vi "Frameremap.vi"(8 "FH":dbl, 9 "FW":dbl, 10 "FO Z":dbl, 11 "FO X":dbl) -> (0 "FH":dbl, 1 "FW":dbl, 2 "Z Origin":dbl, 3 "X Origin":dbl)   [LabVIEW 2019]
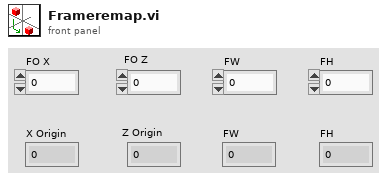
[diagram p1: front panel]
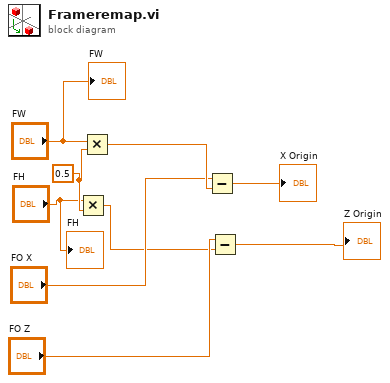
[diagram p0: block diagram]
diagram:
  w9 = 0.5 ("y")
  n1 = Multiply(x="FH", y=w9) -> (x*y=w5:dbl)
  n2 = Multiply(x="FW", y=w9) -> (x*y=w8:dbl)
  n3 = Subtract(x="FO X", y=w8) -> (x-y=→"X Origin":dbl)
  n4 = Subtract(x="FO Z", y=w5) -> (x-y=→"Z Origin":dbl)
  "FW" <- "FW"
  "FH" <- "FH"
